vi "Apply_RF.vi"(0 "I- index":dbl, 4 "I+ index":dbl, 5 "RF Proportional to intensity":bool, 6 "RF Target Position":i32, 7 "RF indicator":bool, 8 "RF Power":dbl, 9 "rho0":dbl[](array[numeric]), 10 "rho-":dbl[](array[numeric]), 11 "rho+":dbl[](array[numeric])) -> (1 "rho- out":dbl[](array[numeric]), 2 "rho0 out":dbl[](array[numeric]), 3 "rho+ out":dbl[](array[numeric]))   [LabVIEW 2018]
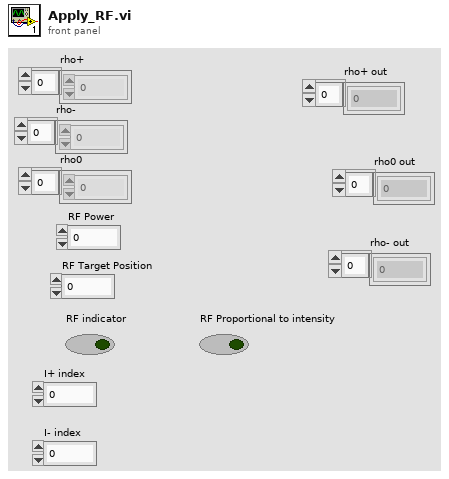
[diagram p1: front panel]
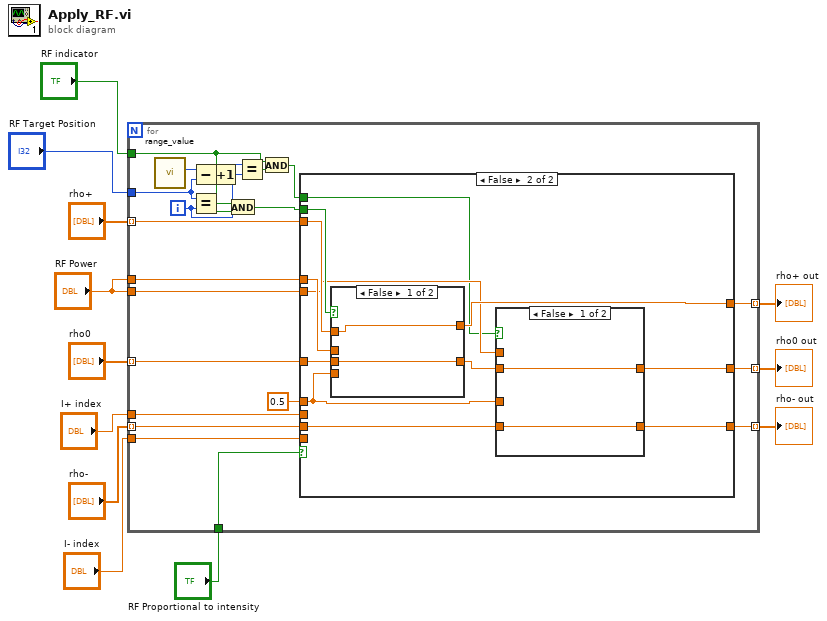
[diagram p0: block diagram]
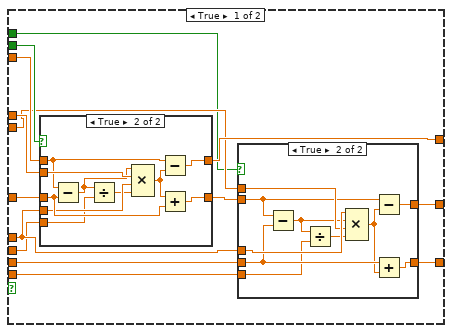
[diagram p2: hidden frame]
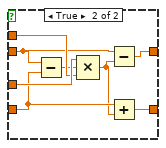
[diagram p5: hidden frame]
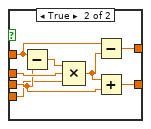
[diagram p6: hidden frame]
diagram:
  n1 = for {
    tunnel: "rho+" -> [w34] mode=indexing
    tunnel: "rho0" -> [w26] mode=indexing
    tunnel: "rho-" -> [w27] mode=indexing
    tunnel: "RF Power" -> [w31]
    tunnel: "RF Target Position" -> [w22]
    tunnel: [w32] -> w8 mode=indexing
    tunnel: [w24] -> w7 mode=indexing
    tunnel: [w29] -> w6 mode=indexing
    tunnel: "RF indicator" -> [w18]
    tunnel: "RF Power" -> [w28]
    tunnel: "I+ index" -> [w16]
    tunnel: "I- index" -> [w15]
    tunnel: "RF Proportional to intensity" -> [w14]
    i -> [w20]
    n2 = call "range_value.vi"() -> ("NumBins"=w23:i32)  [unwired: 10 in, 1 out]
    n3 = Subtract(x=w23, y=w22) -> (x-y=w21:i32)
    n4 = Equal?(x=w22, y=w20) -> (x = y?=w33:bool)
    n5 = Increment(x=w21) -> (x+1=w13:i32)
    n6 = And(x=w33, y=w18) -> (x .and. y?=w30:bool)
    n7 = Equal?(x=w20, y=w13) -> (x = y?=w19:bool)
    n8 = And(x=w18, y=w19) -> (x .and. y?=w17:bool)
    n9 = case shown="False" w14 {
      tunnel: w34 -> [w48 w84]
      tunnel: [w47 w83] -> w32
      tunnel: w31 -> [w46 w82]
      tunnel: w30 -> [w45 w81]
      tunnel: [w44 w80] -> w29
      tunnel: w28 -> [w43 w79]
      tunnel: w27 -> [w42 w78]
      tunnel: w26 -> [w41 w77]
      tunnel: 0.5 -> [w40 w76]
      tunnel: [w38 w74] -> w24
      tunnel: w17 -> [w37 w73]
      tunnel: w16 -> [w36 _]
      tunnel: w15 -> [w35 _]
      frame True {
        n10 = case shown="True" w45 {
          tunnel: w48 -> [w62 w70]
          tunnel: w41 -> [w61 w67]
          tunnel: [w62 w69] -> w47
          tunnel: [w61 w68] -> w39
          tunnel: w46 -> [_ w72]
          tunnel: w40 -> [_ w66]
          tunnel: w36 -> [_ w64]
          frame False {
          }
          frame True {
            n11 = Subtract(x=w70, y=w67) -> (x-y=w63:dbl)
            n12 = Divide(x=w63, y=w64) -> (x/y=w65:dbl)
            n13 = Compound Arithmetic op=MULTIPLY(w63, w72, w66, w65) -> (w71:dbl)
            n14 = Subtract(x=w70, y=w71) -> (x-y=w69:dbl)
            n15 = Add(x=w71, y=w67) -> (x+y=w68:dbl)
          }
        }
        n16 = case shown="True" w37 {
          tunnel: [w49 w60] -> w44
          tunnel: w40 -> [_ w59]
          tunnel: w43 -> [_ w58]
          tunnel: w42 -> [w49 w57]
          tunnel: w39 -> [w50 w55]
          tunnel: [w50 w54] -> w38
          tunnel: w35 -> [_ w51]
          frame False {
          }
          frame True {
            n17 = Subtract(x=w55, y=w57) -> (x-y=w52:dbl)
            n18 = Divide(x=w52, y=w51) -> (x/y=w53:dbl)
            n19 = Compound Arithmetic op=MULTIPLY(w59, w52, w58, w53) -> (w56:dbl)
            n20 = Subtract(x=w55, y=w56) -> (x-y=w54:dbl)
            n21 = Add(x=w57, y=w56) -> (x+y=w60:dbl)
          }
        }
      }
      frame False {
        n22 = case shown="False" w81 {
          tunnel: w84 -> [w96 w101]
          tunnel: w77 -> [w95 w98]
          tunnel: [w96 w100] -> w83
          tunnel: [w95 w99] -> w75
          tunnel: w82 -> [_ w103]
          tunnel: w76 -> [_ w97]
          frame False {
          }
          frame True {
            n23 = Subtract(x=w101, y=w98) -> (x-y=w104:dbl)
            n24 = Compound Arithmetic op=MULTIPLY(w104, w103, w97) -> (w102:dbl)
            n25 = Subtract(x=w101, y=w102) -> (x-y=w100:dbl)
            n26 = Add(x=w102, y=w98) -> (x+y=w99:dbl)
          }
        }
        n27 = case shown="False" w73 {
          tunnel: [w85 w94] -> w80
          tunnel: w76 -> [_ w93]
          tunnel: w79 -> [_ w92]
          tunnel: w78 -> [w85 w90]
          tunnel: w75 -> [w86 w88]
          tunnel: [w86 w87] -> w74
          frame False {
          }
          frame True {
            n28 = Subtract(x=w88, y=w90) -> (x-y=w91:dbl)
            n29 = Compound Arithmetic op=MULTIPLY(w93, w91, w92) -> (w89:dbl)
            n30 = Subtract(x=w88, y=w89) -> (x-y=w87:dbl)
            n31 = Add(x=w90, y=w89) -> (x+y=w94:dbl)
          }
        }
      }
    }
  }
  "rho+ out" <- w8
  "rho0 out" <- w7
  "rho- out" <- w6
